vi "MultiJoint first back.vi"() -> ()   [LabVIEW 2020]
panel:
  in  "Horizontal Pointer Slide 5":dbl(slide) scale=0.0..180.0
  in  "Horizontal Pointer Slide 4":dbl(slide) scale=0.0..180.0
  in  "Horizontal Pointer Slide 3":dbl(slide) scale=0.0..180.0
  in  "Horizontal Pointer Slide 2":dbl(slide) scale=0.0..180.0
  in  "Horizontal Pointer Slide":dbl(slide) scale=0.0..180.0
  out "XY Graph":cluster{dbl[], dbl[]}(graph)
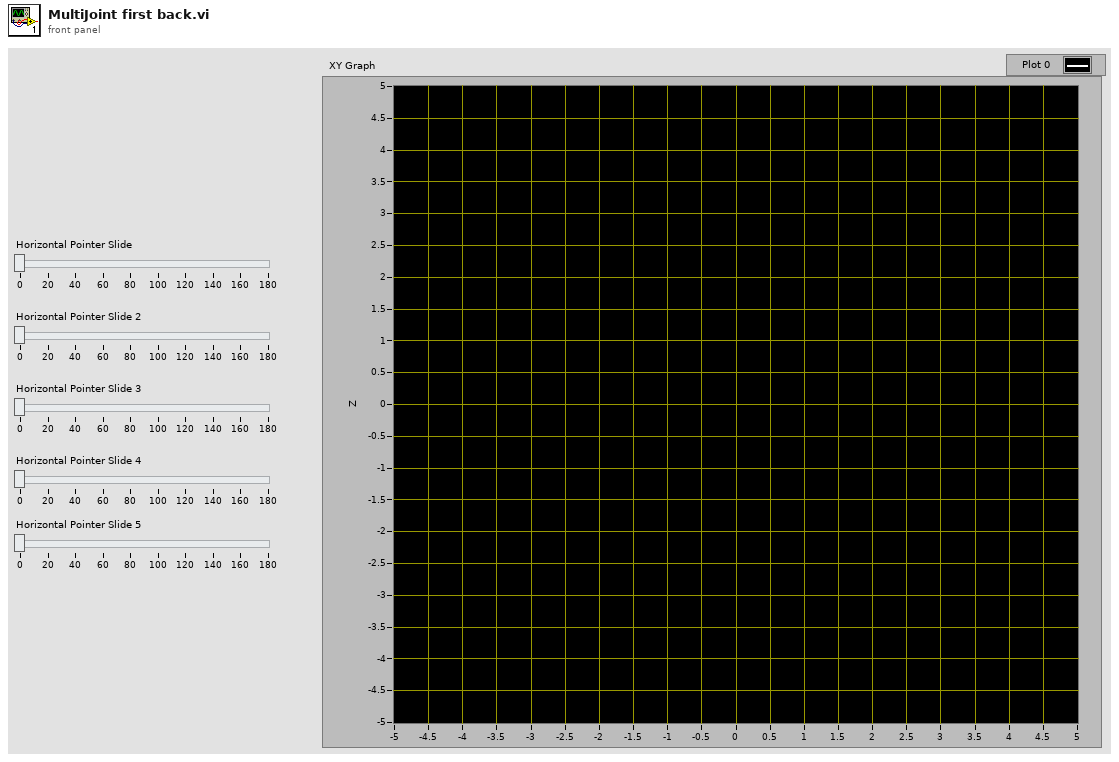
[diagram p1: front panel]
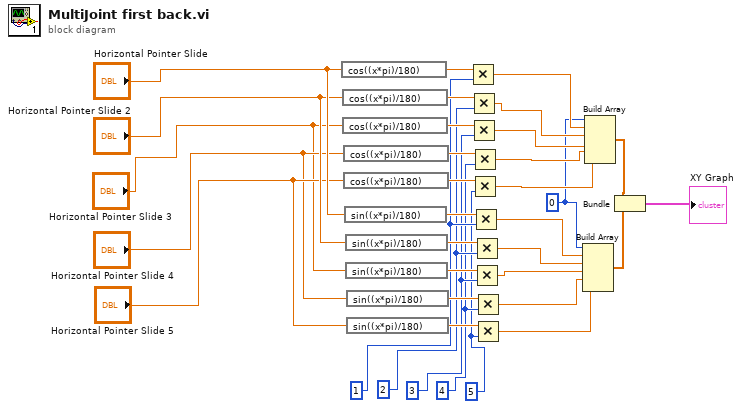
[diagram p0: block diagram]
diagram:
  w6 = 5
  w7 = 4
  w8 = 3
  w9 = 2
  w10 = 1
  w11 = 0
  n1 = expression code="cos((x*pi)/180)"("Horizontal Pointer Slide") -> (w31:dbl)
  n2 = expression code="cos((x*pi)/180)"("Horizontal Pointer Slide 2") -> (w30:dbl)
  n3 = expression code="cos((x*pi)/180)"("Horizontal Pointer Slide 3") -> (w29:dbl)
  n4 = expression code="cos((x*pi)/180)"("Horizontal Pointer Slide 4") -> (w28:dbl)
  n5 = expression code="cos((x*pi)/180)"("Horizontal Pointer Slide 5") -> (w27:dbl)
  n6 = expression code="sin((x*pi)/180)"("Horizontal Pointer Slide") -> (w21:dbl)
  n7 = expression code="sin((x*pi)/180)"("Horizontal Pointer Slide 2") -> (w20:dbl)
  n8 = expression code="sin((x*pi)/180)"("Horizontal Pointer Slide 3") -> (w19:dbl)
  n9 = expression code="sin((x*pi)/180)"("Horizontal Pointer Slide 4") -> (w18:dbl)
  n10 = expression code="sin((x*pi)/180)"("Horizontal Pointer Slide 5") -> (w17:dbl)
  n11 = Multiply(x=w31, y=w10) -> (x*y=w26:dbl)
  n12 = Multiply(x=w30, y=w9) -> (x*y=w25:dbl)
  n13 = Multiply(x=w29, y=w8) -> (x*y=w24:dbl)
  n14 = Multiply(x=w28, y=w7) -> (x*y=w23:dbl)
  n15 = Multiply(x=w27, y=w6) -> (x*y=w22:dbl)
  n16 = Multiply(x=w21, y=w10) -> (x*y=w16:dbl)
  n17 = Multiply(x=w20, y=w9) -> (x*y=w15:dbl)
  n18 = Multiply(x=w19, y=w8) -> (x*y=w14:dbl)
  n19 = Multiply(x=w18, y=w7) -> (x*y=w13:dbl)
  n20 = Multiply(x=w17, y=w6) -> (x*y=w12:dbl)
  n21 = Build Array(w11, w16, w15, w14, w13, w12) -> (w32:dbl[])
  n22 = Build Array(w11, w26, w25, w24, w23, w22) -> (w33:dbl[])
  n23 = Bundle(w33, w32) -> (→"XY Graph":cluster{dbl[], dbl[]})  [unwired: 1 in]
